vi "ALTS-2015 Simulate Write Result DB.vi"(8 "error in":errorcluster, 11 "Simulate Result DB Path":path) -> (0 "error out":errorcluster)   [LabVIEW 2013]
uses:
  <vilib>/Utility/file.llb/Write To Spreadsheet File (string).vi
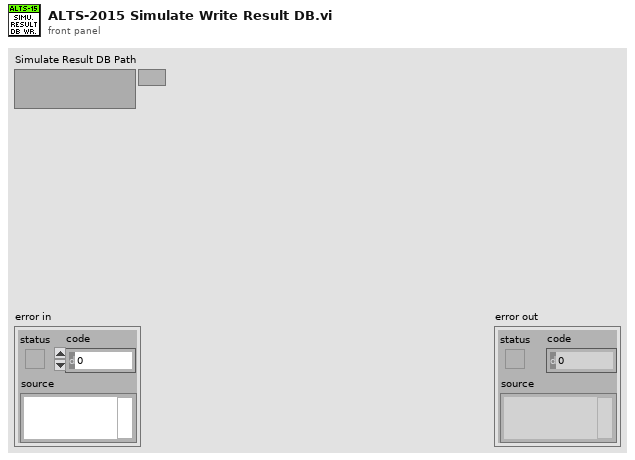
[diagram p1: front panel]
types:
  T1 = typedef "ALTS-2015 DB Result Cluster.ctl" = cluster{"Sensor_Name":string, "SN":string, "Work_order_Number":string, "User1":string, "User2":string, "User3":string, "User4":string, "Pressure":dbl, "Flow":dbl, "Test_Result":string, "Test_Time":string}
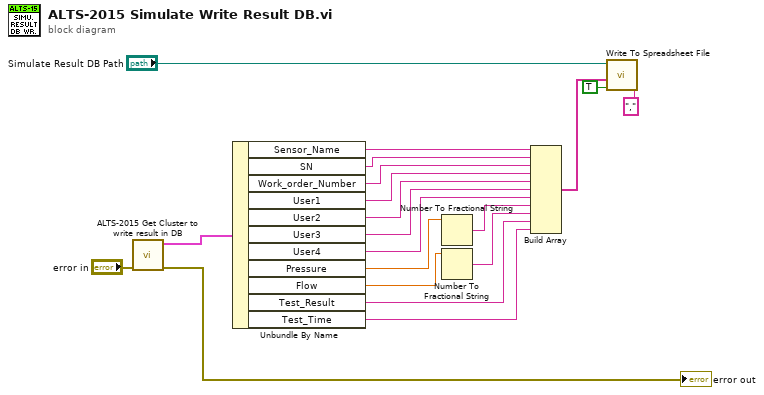
[diagram p0: block diagram]
diagram:
  n1 = call "ALTS-2015 Get Cluster to write result in DB.vi"("error in"="error in") -> ("error out"=→"error out":errorcluster, "DB Result Cluster Out"=w19:T1)  [unwired: 9 in]
  n2 = Unbundle By Name(w19) -> ("Sensor_Name"=w2:string, "SN"=w14:string, "Work_order_Number"=w13:string, "User1"=w12:string, "User2"=w11:string, "User3"=w10:string, "User4"=w9:string, "Pressure"=w16:dbl, "Flow"=w15:dbl, "Test_Result"=w6:string, "Test_Time"=w5:string)
  n3 = Number To Fractional String(number=w16) -> (F-format string=w8:string)  [unwired: 3 in]
  n4 = Number To Fractional String(number=w15) -> (F-format string=w7:string)  [unwired: 3 in]
  n5 = Build Array(w2, w14, w13, w12, w11, w10, w9, w8, w7, w6, w5) -> (w4:string[])
  n6 = call-poly <vilib>:"Write To Spreadsheet File.vi"("delimiter (\\t)"="," ("delimiter (\\t)"), "append to file? (new file:F)"=TRUE, "1D data"=w4, "file path (dialog if empty)"="Simulate Result DB Path") -> ()  [unwired: 4 in, 1 out]
